vi "RearrangeCasesAlphabetically.vi"(8 "error in (no error)":errorcluster, 11 "CaseStructure Ref":refnum<vi>) -> (0 "error out":errorcluster, 3 "CaseStructure Ref":refnum<vi>)   [LabVIEW 2019, in "BlueUtilityScripts.lvlib"]
uses:
  BlueUtilityScripts.lvlib
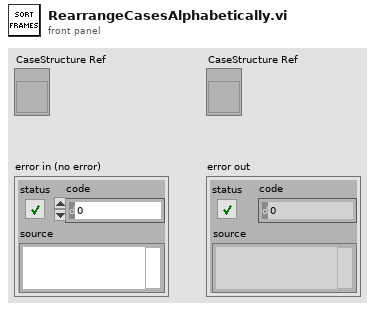
[diagram p1: front panel]
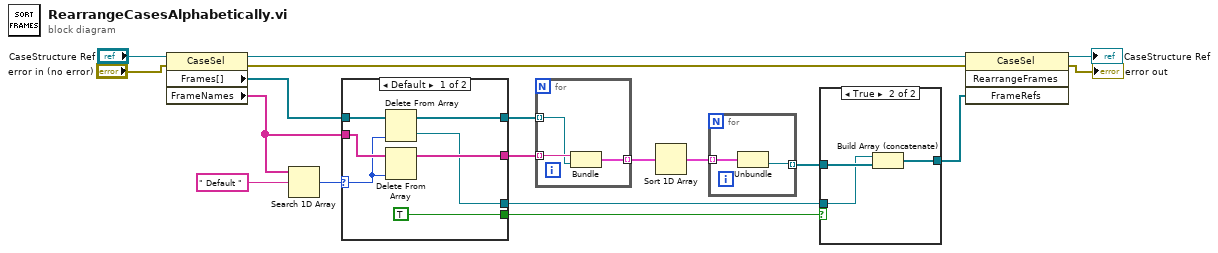
[diagram p0: block diagram]
diagram:
  n1 = property class="CaseSel"(reference="CaseStructure Ref", error in="error in (no error)") -> (reference out=w11:refnum<vi>, error out=w6:errorcluster, "Frames[]"=w16:refnum<vi>[], "FrameNames"=w17:string[])
  n2 = Search 1D Array(1D array=w17, element=" Default ") -> (index of element=w12:i32)  [unwired: 1 in]
  n3 = case shown="Default" w12 {
    selector: w12 -> [w23 _]
    tunnel: w17 -> [w24 w26]
    tunnel: w16 -> [w25 w27]
    tunnel: [w22 w27] -> w15
    tunnel: [w21 w26] -> w14
    tunnel: [TRUE _] -> w4
    tunnel: [w19 _] -> w2
    frame Default {
      n4 = Delete From Array(array=w25, index=w23) -> (deleted portion=w19:refnum<vi>, array with subset deleted=w22:refnum<vi>[])  [unwired: 1 in]
      n5 = Delete From Array(array=w24, index=w23) -> (array with subset deleted=w21:string[])  [unwired: 1 in, 1 out]
    }
    frame -1 {
    }
  }
  n6 = for {
    tunnel: w15 -> [w29] mode=indexing
    tunnel: w14 -> [w30] mode=indexing
    tunnel: [w28] -> w13 mode=indexing
    n7 = Bundle(w30, w29) -> (w28:cluster{string, refnum<vi>})  [unwired: 1 in]
  }
  n8 = Sort 1D Array(array=w13) -> (sorted array=w5:cluster{string, refnum<vi>}[])
  n9 = for {
    tunnel: w5 -> [w32] mode=indexing
    tunnel: [w31] -> w3 mode=indexing
    n10 = Unbundle(w32) -> (w31:refnum<vi>)  [unwired: 1 out]
  }
  n11 = case shown="True" w4 {
    tunnel: w3 -> [w33 w36]
    tunnel: w2 -> [_ w35]
    tunnel: [w33 w34] -> w1
    frame False {
    }
    frame True {
      n12 = Build Array (concatenate)(w35, w36) -> (w34:refnum<vi>[])
    }
  }
  n13 = invoke class="CaseSel" method="RearrangeFrames"(reference=w11, error in=w6, "FrameRefs"=w1) -> (reference out=→"CaseStructure Ref":refnum<vi>, error out=→"error out":errorcluster)  [unwired: 1 in, 2 out]
